vi "final.vi"() -> ()   [LabVIEW 2015]
uses:
  <vilib>/NXT/Block Support/NXT_InputPort.ctl
  <vilib>/NXT/Subs/MotorOutput.ctl
  <vilib>/NXT/Dual Mode Library/Sensors/Sonar_cm.vi
  <vilib>/NXT/Dual Mode Library/Sensors/Light_On.vi
  <vilib>/NXT/Dual Mode Library/Motors/MotorReverse.vi
  <vilib>/NXT/Dual Mode Library/Waits/Wait_Num.vi
  <vilib>/NXT/Dual Mode Library/Motors/MotorOn.vi
panel:
  in  "沥瘤":bool
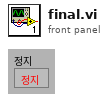
[diagram p1: front panel]
types:
  T1 = typedef "MotorOutput.ctl" = u8
  T2 = typedef "NXT_InputPort.ctl" = u32
  T3 = typedef "LVHSConnector.ctl" = refnum<class "BrickReference.lvclass">
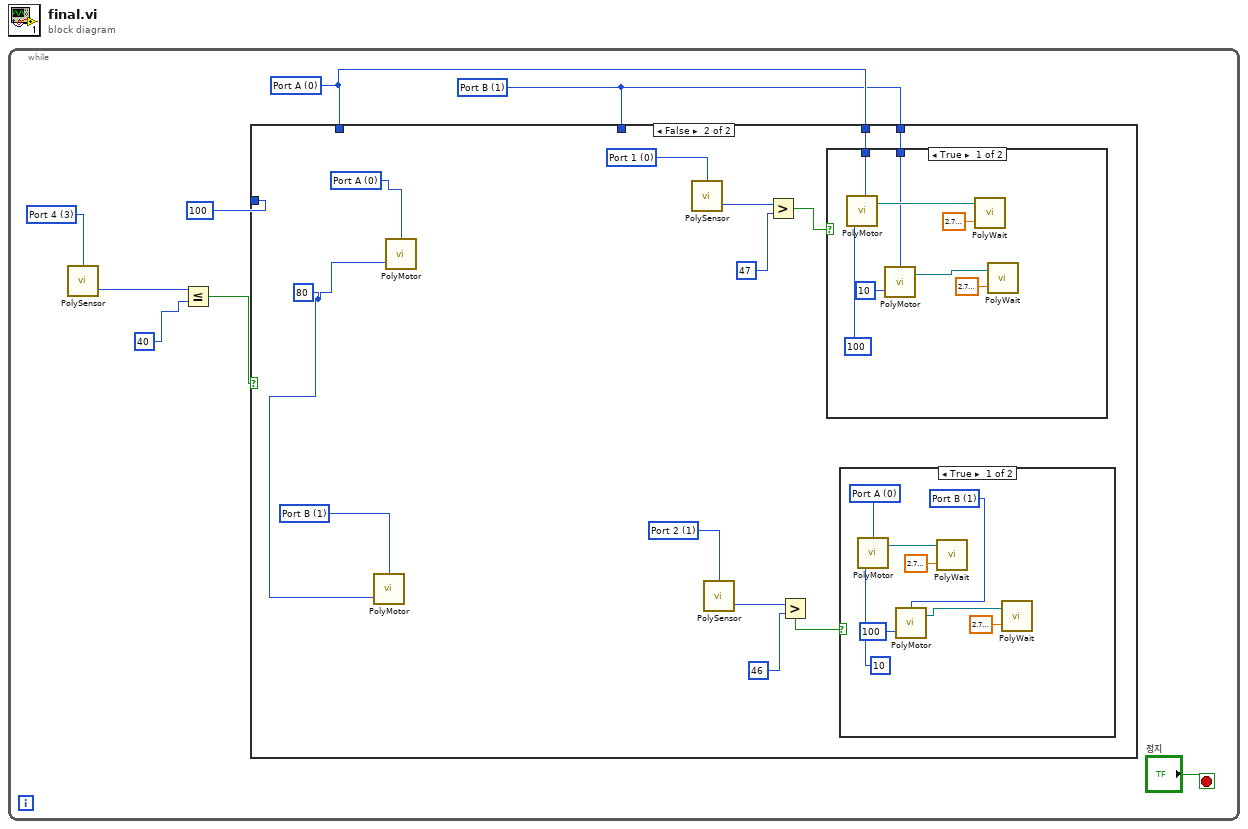
[diagram p0: block diagram]
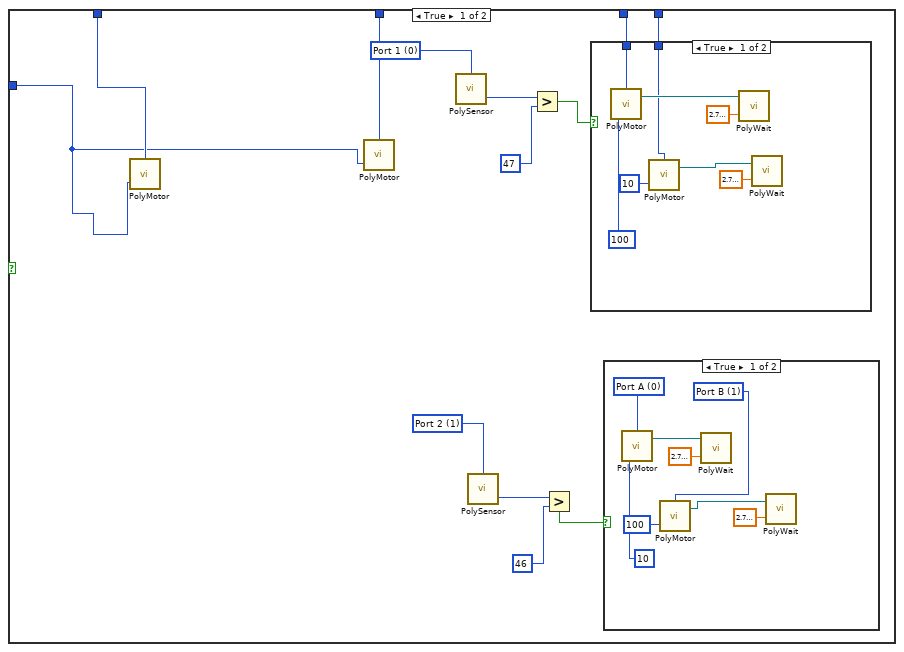
[diagram p2: hidden frame]
diagram:
  n1 = while {
    stop <- "沥瘤" stop-if-true
    w1 = T1 1 items=["Port A", "Port B", "Port C", "All Ports"] ("Output Port (All Ports)")
    w2 = T1 0 items=["Port A", "Port B", "Port C", "All Ports"] ("Output Port (All Ports)")
    w5 = T2 3 items=["Port 1", "Port 2", "Port 3", "Port 4"] ("Input Port")
    n2 = call-poly <vilib>:"PolySensor.vi"("Port (Port 4)"=w5) -> ("Distance (cm)"=w3:i16)  [unwired: 2 in, 1 out]
    n3 = Less Or Equal?(x=w3, y=40) -> (x <= y?=w6:bool)
    n4 = case shown="False" w6 {
      tunnel: w2 -> [w21 _]
      tunnel: 100 ("Power (75)") -> [w19 _]
      tunnel: w1 -> [w20 _]
      tunnel: w2 -> [w10 w41]
      tunnel: w1 -> [w9 w40]
      frame True {
        w12 = T2 1 items=["Port 1", "Port 2", "Port 3", "Port 4"] ("Input Port")
        w11 = T2 0 items=["Port 1", "Port 2", "Port 3", "Port 4"] ("Input Port")
        n5 = call-poly <vilib>:"PolyMotor.vi"("Power (75)"=w19, "Output Port (All Ports)"=w21) -> ()  [unwired: 2 in, 1 out]
        n6 = call-poly <vilib>:"PolyMotor.vi"("Power (75)"=w19, "Output Port (All Ports)"=w20) -> ()  [unwired: 2 in, 1 out]
        n7 = call-poly <vilib>:"PolySensor.vi"("Port (Port 3)"=w11) -> ("Scaled Value"=w15:i16)  [unwired: 2 in, 1 out]
        n8 = call-poly <vilib>:"PolySensor.vi"("Port (Port 3)"=w12) -> ("Scaled Value"=w18:i16)  [unwired: 2 in, 1 out]
        n9 = Greater?(x=w15, y=47) -> (0:w13:bool)
        n10 = Greater?(x=w18, y=46) -> (0:w16:bool)
        n11 = case shown="True" w13 {
          tunnel: w10 -> [w23 _]
          tunnel: w9 -> [w22 _]
          frame True {
            n12 = call-poly <vilib>:"PolyMotor.vi"("Power (75)"=100, "Output Port (All Ports)"=w23) -> ("NXT/EV3"=w29:T3)  [unwired: 2 in]
            n13 = call-poly <vilib>:"PolyMotor.vi"("Power (75)"=10, "Output Port (All Ports)"=w22) -> ("NXT/EV3"=w26:T3)  [unwired: 2 in]
            n14 = call-poly <vilib>:"PolyWait.vi"("Time (1 sec)"=sgl 2.7 ("Time (sec)"), "NXT/EV3"=w29) -> ()  [unwired: 2 in, 1 out]
            n15 = call-poly <vilib>:"PolyWait.vi"("Time (1 sec)"=sgl 2.7 ("Time (sec)"), "NXT/EV3"=w26) -> ()  [unwired: 2 in, 1 out]
          }
          frame False {
          }
        }
        n16 = case shown="True" w16 {
          frame True {
            w32 = T1 1 items=["Port A", "Port B", "Port C", "All Ports"] ("Output Port (All Ports)")
            w35 = T1 0 items=["Port A", "Port B", "Port C", "All Ports"] ("Output Port (All Ports)")
            n17 = call-poly <vilib>:"PolyMotor.vi"("Power (75)"=10, "Output Port (All Ports)"=w35) -> ("NXT/EV3"=w37:T3)  [unwired: 2 in]
            n18 = call-poly <vilib>:"PolyMotor.vi"("Power (75)"=100, "Output Port (All Ports)"=w32) -> ("NXT/EV3"=w33:T3)  [unwired: 2 in]
            n19 = call-poly <vilib>:"PolyWait.vi"("Time (1 sec)"=sgl 2.7 ("Time (sec)"), "NXT/EV3"=w37) -> ()  [unwired: 2 in, 1 out]
            n20 = call-poly <vilib>:"PolyWait.vi"("Time (1 sec)"=sgl 2.7 ("Time (sec)"), "NXT/EV3"=w33) -> ()  [unwired: 2 in, 1 out]
          }
          frame False {
          }
        }
      }
      frame False {
        w39 = T1 1 items=["Port A", "Port B", "Port C", "All Ports"] ("Output Port (All Ports)")
        w43 = T2 1 items=["Port 1", "Port 2", "Port 3", "Port 4"] ("Input Port")
        w42 = T2 0 items=["Port 1", "Port 2", "Port 3", "Port 4"] ("Input Port")
        w38 = 80 ("Power (75)")
        w50 = T1 0 items=["Port A", "Port B", "Port C", "All Ports"] ("Output Port (All Ports)")
        n21 = call-poly <vilib>:"PolyMotor.vi"("Power (75)"=w38, "Output Port (All Ports)"=w39) -> ()  [unwired: 2 in, 1 out]
        n22 = call-poly <vilib>:"PolyMotor.vi"("Power (75)"=w38, "Output Port (All Ports)"=w50) -> ()  [unwired: 2 in, 1 out]
        n23 = call-poly <vilib>:"PolySensor.vi"("Port (Port 3)"=w42) -> ("Scaled Value"=w46:i16)  [unwired: 2 in, 1 out]
        n24 = call-poly <vilib>:"PolySensor.vi"("Port (Port 3)"=w43) -> ("Scaled Value"=w49:i16)  [unwired: 2 in, 1 out]
        n25 = Greater?(x=w46, y=47) -> (0:w44:bool)
        n26 = Greater?(x=w49, y=46) -> (0:w47:bool)
        n27 = case shown="True" w44 {
          tunnel: w41 -> [w56 _]
          tunnel: w40 -> [w52 _]
          frame True {
            n28 = call-poly <vilib>:"PolyMotor.vi"("Power (75)"=100, "Output Port (All Ports)"=w56) -> ("NXT/EV3"=w58:T3)  [unwired: 2 in]
            n29 = call-poly <vilib>:"PolyMotor.vi"("Power (75)"=10, "Output Port (All Ports)"=w52) -> ("NXT/EV3"=w54:T3)  [unwired: 2 in]
            n30 = call-poly <vilib>:"PolyWait.vi"("Time (1 sec)"=sgl 2.7 ("Time (sec)"), "NXT/EV3"=w58) -> ()  [unwired: 2 in, 1 out]
            n31 = call-poly <vilib>:"PolyWait.vi"("Time (1 sec)"=sgl 2.7 ("Time (sec)"), "NXT/EV3"=w54) -> ()  [unwired: 2 in, 1 out]
          }
          frame False {
          }
        }
        n32 = case shown="True" w47 {
          frame True {
            w61 = T1 1 items=["Port A", "Port B", "Port C", "All Ports"] ("Output Port (All Ports)")
            w64 = T1 0 items=["Port A", "Port B", "Port C", "All Ports"] ("Output Port (All Ports)")
            n33 = call-poly <vilib>:"PolyMotor.vi"("Power (75)"=10, "Output Port (All Ports)"=w64) -> ("NXT/EV3"=w66:T3)  [unwired: 2 in]
            n34 = call-poly <vilib>:"PolyMotor.vi"("Power (75)"=100, "Output Port (All Ports)"=w61) -> ("NXT/EV3"=w62:T3)  [unwired: 2 in]
            n35 = call-poly <vilib>:"PolyWait.vi"("Time (1 sec)"=sgl 2.7 ("Time (sec)"), "NXT/EV3"=w66) -> ()  [unwired: 2 in, 1 out]
            n36 = call-poly <vilib>:"PolyWait.vi"("Time (1 sec)"=sgl 2.7 ("Time (sec)"), "NXT/EV3"=w62) -> ()  [unwired: 2 in, 1 out]
          }
          frame False {
          }
        }
      }
    }
  }
